vi "Quiz Alt.vi"() -> ()   [LabVIEW 2012]
uses:
  Controls/Quiz Solution.ctl
  Controls/Quiz Question.ctl
  Controls/Problem Type enum.ctl
  Controls/Solution Type enum.ctl
  Controls/Quiz Set Up.ctl
panel:
  in  "Question Array Out":T1[](array[typedef])=[{"Text"="\"Enter \"\"AAA\"\"\"", "Problem Type"=enum."Text", "Solution Type"=enum."Text", "Picture"=bytes[0], "MultiText"=[], "Solution"={"Answer State"=enum."Unanswered", "TF Answer"=enum."No Selection", "Text Answer"="AAA", "Multi Answer"=[], "ExactMatch"=TRUE, "Numeric Answer"={"NumAnswer"=0.0, "Num Sol MAX"=0.0, "Num Sol MIN"=0.0, "SigFig?"=FALSE, "Num Sig Figs"=0}, "T/F_Solution"=FALSE}}, {"Text"="Which one is conductive", "Problem Type"=enum."Text&Image", "Solution Type"=enum."SelectOne", "Picture"=bytes[117294], "MultiText"=["AA", "BB", "CC"], "Solution"={"Answer State"=enum."Unanswered", "TF Answer"=enum."No Selection", "Text Answer"="", "Multi Answer"=[FALSE, TRUE, FALSE], "ExactMatch"=FALSE, "Numeric Answer"={"NumAnswer"=0.0, "Num Sol MAX"=0.0, "Num Sol MIN"=0.0, "SigFig?"=FALSE, "Num Sig Figs"=0}, "T/F_Solution"=FALSE}}, {"Text"="Select the Vowels", "Problem Type"=enum."Text", "Solution Type"=enum."SelectMultiple", "Picture"=bytes[0], "MultiText"=["A'", "B'", "E'", "D'", "U'"], "Solution"={"Answer State"=enum."Unanswered", "TF Answer"=enum."No Selection", "Text Answer"="", "Multi Answer"=[TRUE, FALSE, TRUE, FALSE, TRUE], "ExactMatch"=FALSE, "Numeric Answer"={"NumAnswer"=0.0, "Num Sol MAX"=0.0, "Num Sol MIN"=0.0, "SigFig?"=FALSE, "Num Sig Figs"=0}, "T/F_Solution"=FALSE}}, {"Text"="Select True", "Problem Type"=enum."Text", "Solution Type"=enum."True/False", "Picture"=bytes[0], "MultiText"=[], "Solution"={"Answer State"=enum."Unanswered", "TF Answer"=enum."No Selection", "Text Answer"="", "Multi Answer"=[], "ExactMatch"=FALSE, "Numeric Answer"={"NumAnswer"=0.0, "Num Sol MAX"=0.0, "Num Sol MIN"=0.0, "SigFig?"=FALSE, "Num Sig Figs"=0}, "T/F_Solution"=TRUE}}, {"Text"="8<x<10 (3 sig figs)", "Problem Type"=enum."Text&Image", "Solution Type"=enum."Numeric", "Picture"=bytes[107210], "MultiText"=[], "Solution"={"Answer State"=enum."Unanswered", "TF Answer"=enum."No Selection", "Text Answer"="", "Multi Answer"=[], "ExactMatch"=FALSE, "Numeric Answer"={"NumAnswer"=0.0, "Num Sol MAX"=0.0, "Num Sol MIN"=8.0, "SigFig?"=TRUE, "Num Sig Figs"=3}, "T/F_Solution"=FALSE}}]
  in  "Problem2":T4={"ProblemNum"=0, "Problem Type"={"Text"="", "Image"=bytes[0], "Text&Image"={"Text (&Image)"="", "Image (&text)"=bytes[0]}}, "Solution Type"={"Numeric"=0.0, "String"="", "Multi"={"A"=FALSE, "B"=FALSE, "C"=FALSE, "D"=FALSE, "E"=TRUE}, "Radio"=enum."E", "True/False"=enum."True", "Short Answer"=""}, "Answer Color"=0, "Submit"=FALSE}
  in  "Problem1":T4={"ProblemNum"=0, "Problem Type"={"Text"="", "Image"=bytes[0], "Text&Image"={"Text (&Image)"="", "Image (&text)"=bytes[0]}}, "Solution Type"={"Numeric"=0.0, "String"="", "Multi"={"A"=FALSE, "B"=FALSE, "C"=FALSE, "D"=FALSE, "E"=TRUE}, "Radio"=enum."E", "True/False"=enum."True", "Short Answer"=""}, "Answer Color"=0, "Submit"=FALSE}
  in  "Problem0":T4={"ProblemNum"=0, "Problem Type"={"Text"="", "Image"=bytes[0], "Text&Image"={"Text (&Image)"="", "Image (&text)"=bytes[0]}}, "Solution Type"={"Numeric"=0.0, "String"="", "Multi"={"A"=FALSE, "B"=FALSE, "C"=FALSE, "D"=FALSE, "E"=TRUE}, "Radio"=enum."E", "True/False"=enum."True", "Short Answer"=""}, "Answer Color"=0, "Submit"=FALSE}
  in  "Problem Offset (0)":i32
  in  "? Ref Array":refnum<vi>[](array[refnum])
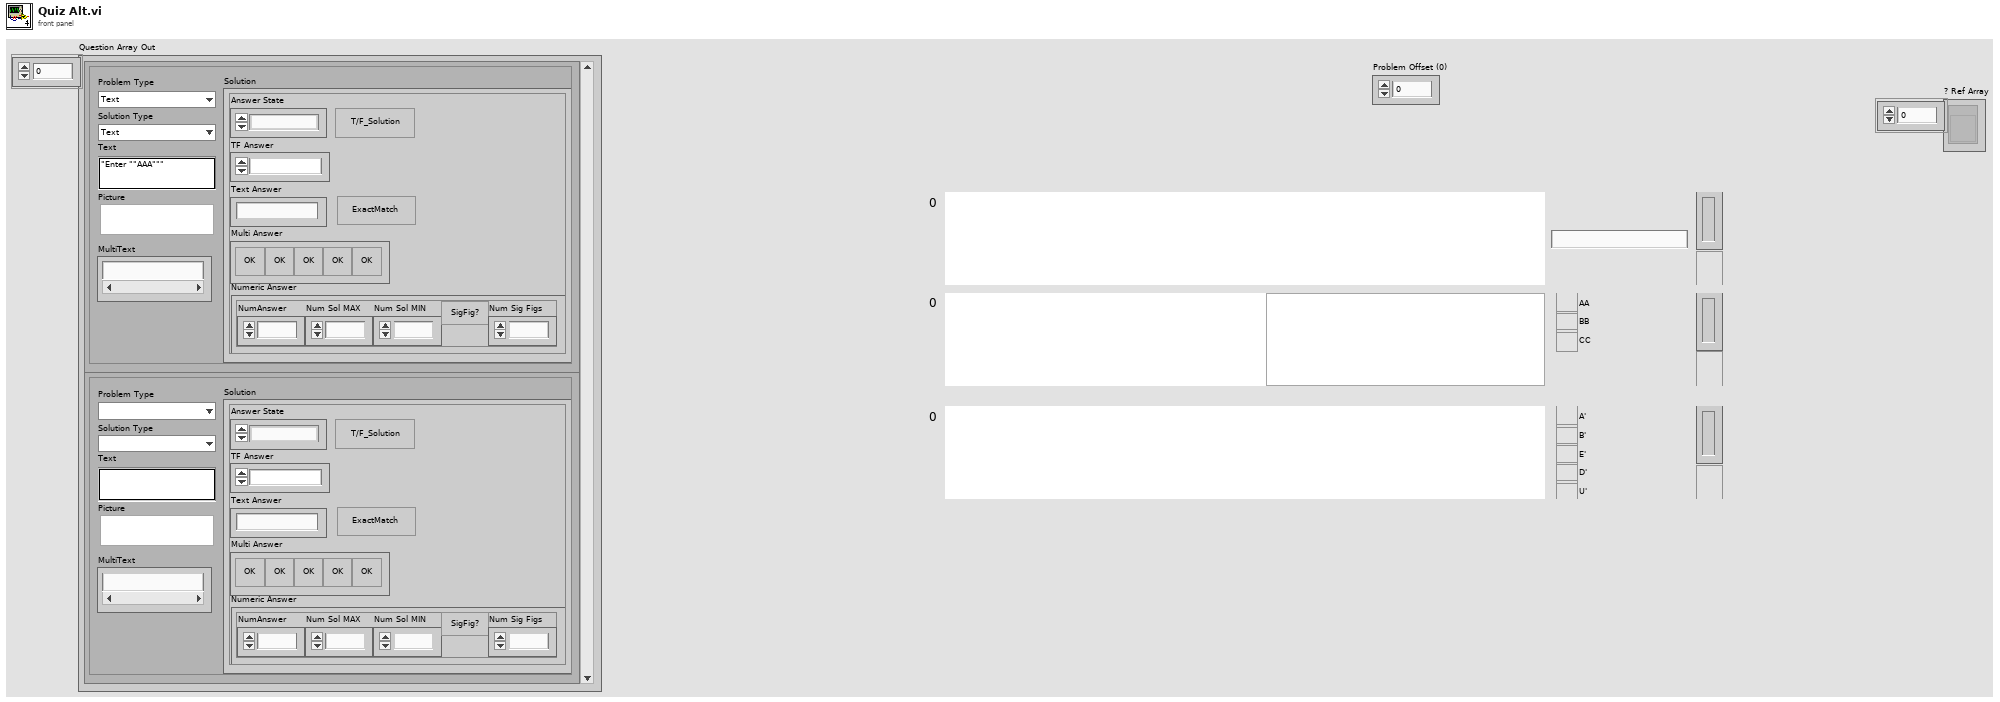
[diagram p1: front panel]
types:
  T1 = typedef "Quiz Set Up.ctl" = cluster{"Text":string, "Problem Type":T2, "Solution Type":T3, "Picture":picture, "MultiText":string[], "Solution":cluster{"Answer State":enum16{"Unanswered", "Correct", "Incorrect"}, "TF Answer":enum32{"No Selection", "True", "False"}, "Text Answer":string, "Multi Answer":bool[], "ExactMatch":bool, "Numeric Answer":cluster{"NumAnswer":dbl, "Num Sol MAX":dbl, "Num Sol MIN":dbl, "SigFig?":bool, "Num Sig Figs":i32}, "T/F_Solution":bool}}
  T2 = typedef "Problem Type enum.ctl" = enum16{"Text", "Image", "Text&Image"}
  T3 = typedef "Solution Type enum.ctl" = enum16{"Numeric", "Text", "SelectMultiple", "SelectOne", "True/False", "ShortAnswer"}
  T4 = typedef "Quiz Question.ctl" = cluster{"ProblemNum":i32, "Problem Type":cluster{"Text":string, "Image":picture, "Text&Image":cluster{"Text (&Image)":string, "Image (&text)":picture}}, "Solution Type":cluster{"Numeric":dbl, "String":string, "Multi":cluster{"A":bool, "B":bool, "C":bool, "D":bool, "E":bool}, "Radio":enum32{"No Selection", "A", "B", "C", "D", "E"}, "True/False":enum32{"No Selection", "True", "False"}, "Short Answer":string}, "Answer Color":u32, "Submit":bool}
  T5 = typedef "Quiz Solution.ctl" = cluster{"Answer State":enum16{"Unanswered", "Correct", "Incorrect"}, "TF Answer":enum32{"No Selection", "True", "False"}, "Text Answer":string, "Multi Answer":bool[], "NumAnswer":dbl}
  T6 = enum8{"Enabled", "Disabled", "Disabled and Grayed Out"}
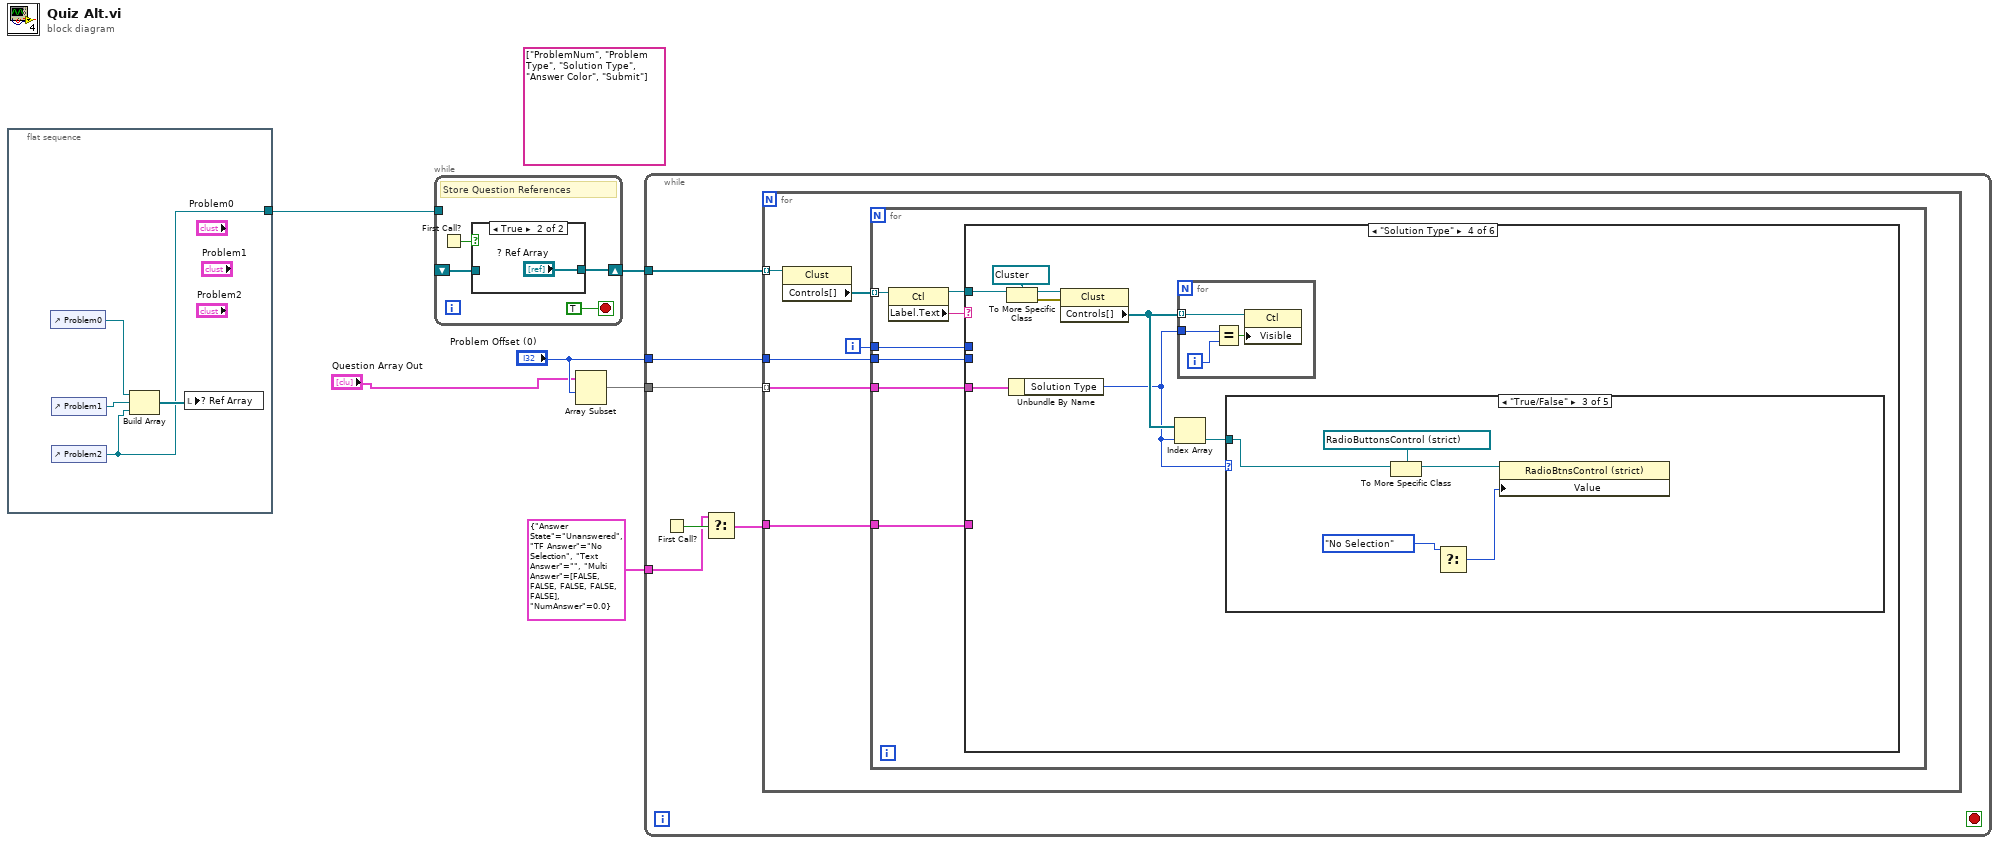
[diagram p0: block diagram]
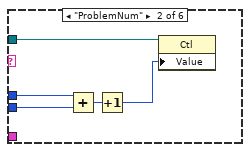
[diagram p3: hidden frame]
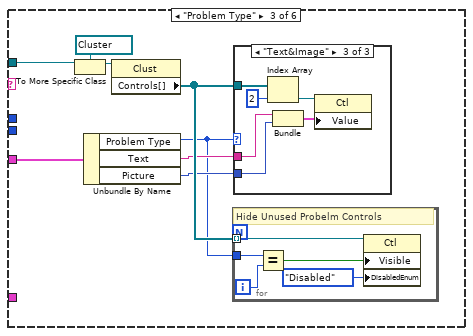
[diagram p4: hidden frame]
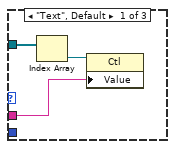
[diagram p5: hidden frame]
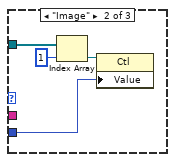
[diagram p6: hidden frame]
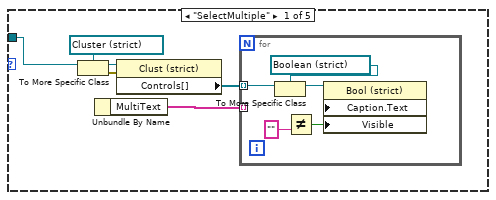
[diagram p7: hidden frame]
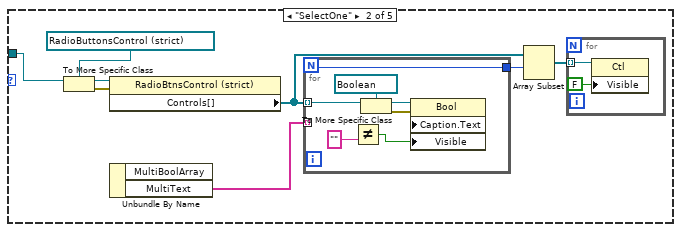
[diagram p8: hidden frame]
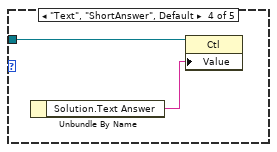
[diagram p9: hidden frame]
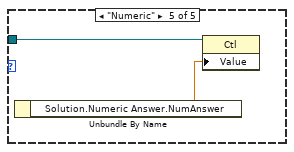
[diagram p10: hidden frame]
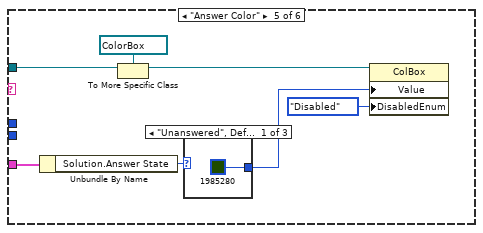
[diagram p11: hidden frame]
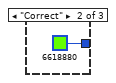
[diagram p12: hidden frame]
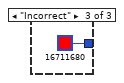
[diagram p13: hidden frame]
diagram:
  (unwired) string[] ["ProblemNum", "Problem Type", "Solution Type", "Answer Color", "Submit"] ("Array")
  n1 = flat-sequence {
    tunnel: [w7] -> w4
    frame #0 {
      n2 = control-ref of="Problem0"() -> (w9:refnum<vi>)
      n3 = control-ref of="Problem1"() -> (w8:refnum<vi>)
      n4 = control-ref of="Problem2"() -> (w7:refnum<vi>)
      n5 = Build Array(w9, w8, w7) -> (w10:refnum<vi>[])
      n6 = local write "? Ref Array"(w10) -> ()
    }
  }
  n7 = while {
    shift-right: [w14] -> w6
    shift-left: _ -> [w13]
    tunnel: w4 -> [_]
    stop <- TRUE stop-if-true
    # "Store Question References"
    n8 = First Call?() -> (First Call?: T/F=w11:bool)
    n9 = case shown="True" w11 {
      tunnel: [w15 "? Ref Array"] -> w14
      tunnel: w13 -> [w15 _]
      frame False {
      }
      frame True {
      }
    }
  }
  n10 = Array Subset(array="Question Array Out", index="Problem Offset (0)") -> (w5:T1[])  [unwired: 1 in]
  n11 = while {
    tunnel: w6 -> [w22]
    tunnel: w5 -> [w21]
    tunnel: "Problem Offset (0)" -> [w20]
    tunnel: T5 {"Answer State"=enum."Unanswered", "TF Answer"=enum."No Selection", "Text Answer"="", "Multi Answer"=[FALSE, FALSE, FALSE, FALSE, FALSE], "NumAnswer"=0.0} ("Solution") -> [w18]
    stop <- _ stop-if-true
    n12 = First Call?() -> (First Call?: T/F=w19:bool)
    n13 = Select(t=w18, s=w19) -> (s? t:f=w17:T5)  [unwired: 1 in]
    n14 = for {
      tunnel: w22 -> [w28] mode=indexing
      tunnel: w21 -> [w24] mode=indexing
      tunnel: w20 -> [w26]
      tunnel: w17 -> [w23]
      i -> [w25]
      n15 = property class="Clust"(reference=w28) -> ("Controls[]"=w27:refnum<vi>[])  [unwired: 1 in, 2 out]
      n16 = for {
        tunnel: w27 -> [w35] mode=indexing
        tunnel: w26 -> [w32]
        tunnel: w25 -> [w31]
        tunnel: w24 -> [w30]
        tunnel: w23 -> [w29]
        n17 = property class="Ctl"(reference=w35) -> (reference out=w33:refnum<vi>, "Label.Text"=w34:string)  [unwired: 1 in, 1 out]
        n18 = case shown="\"Solution Type\"" w34 {
          tunnel: w33 -> [_ w40 w45 w73 w119 _]
          tunnel: w32 -> [_ w38 _ _ _ _]
          tunnel: w31 -> [_ w37 _ _ _ _]
          tunnel: w30 -> [_ _ w48 w67 w122 _]
          tunnel: w29 -> [_ _ _ _ _ _]
          frame "NULL", Default {
          }
          frame "ProblemNum" {
            n19 = Add(x=w37, y=w38) -> (x+y=w39:i32)
            n20 = Increment(x=w39) -> (x+1=w36:i32)
            n21 = property class="Ctl"(reference=w40, "Value"=w36) -> ()  [unwired: 1 in, 2 out]
          }
          frame "Problem Type" {
            n22 = To More Specific Class(target class=refnum<vi> refnum ("Problem Type"), reference=w45) -> (specific class reference=w46:refnum<vi>)  [unwired: 1 in, 1 out]
            n23 = Unbundle By Name(w48) -> ("Problem Type"=w41:T2, "Text"=w43:string, "Picture"=w42:picture)
            n24 = property on="Property Node" class="Clust"(reference=w46) -> ("Controls[]"=w44:refnum<vi>[])  [unwired: 1 in, 2 out]
            n25 = for "Problem Controls" {
              tunnel: w44 -> [w66] mode=indexing
              tunnel: w41 -> [w64]
              i -> [w63]
              # "Hide Unused Probelm Controls"
              n26 = Equal?(x=w64, y=w63) -> (x = y?=w62:bool)
              n27 = property on="Property Node" class="Ctl"(reference=w66, "Visible"=w62, "DisabledEnum"=T6."Disabled" ("Disabled")) -> ()  [unwired: 1 in, 2 out]
            }
            n28 = case shown="\"Text&Image\"" w41 {
              tunnel: w44 -> [w51 w55 w61]
              tunnel: w43 -> [w49 _ w58]
              tunnel: w42 -> [_ w52 w57]
              frame "Text", Default {
                n29 = Index Array(array=w51) -> (element=w50:refnum<vi>)  [unwired: 1 in]
                n30 = property on="Property Node" class="Ctl"(reference=w50, "Value"=w49) -> ()  [unwired: 1 in, 2 out]
              }
              frame "Image" {
                n31 = Index Array(array=w55, index=1) -> (element=w53:refnum<vi>)
                n32 = property on="Property Node" class="Ctl"(reference=w53, "Value"=w52) -> ()  [unwired: 1 in, 2 out]
              }
              frame "Text&Image" {
                n33 = Index Array(array=w61, index=2) -> (element=w59:refnum<vi>)
                n34 = Bundle("Text"=w58, "Picture"=w57) -> (w56:cluster{"Text":string, "Picture":picture})  [unwired: 1 in]
                n35 = property on="Property Node" class="Ctl"(reference=w59, "Value"=w56) -> ()  [unwired: 1 in, 2 out]
              }
            }
          }
          frame "Solution Type" {
            n36 = To More Specific Class(target class=refnum<vi> refnum ("Problem Type"), reference=w73) -> (specific class reference=w72:refnum<vi>, error out=w71:errorcluster)  [unwired: 1 in]
            n37 = Unbundle By Name(w67) -> ("Solution Type"=w69:T3)
            n38 = property on="Property Node" class="Clust"(reference=w72, error in=w71) -> ("Controls[]"=w70:refnum<vi>[])  [unwired: 2 out]
            n39 = Index Array(array=w70, index=w69) -> (element=w68:refnum<vi>)
            n40 = for {
              tunnel: w70 -> [w115] mode=indexing
              tunnel: w69 -> [w113]
              i -> [w112]
              n41 = Equal?(x=w113, y=w112) -> (x = y?=w114:bool)
              n42 = property on="Property Node" class="Ctl"(reference=w115, "Visible"=w114) -> ()  [unwired: 1 in, 2 out]
            }
            n43 = case "Populate Solution Controls" shown="\"True/False\"" w69 {
              tunnel: w68 -> [w75 w86 w105 w109 w110]
              frame "SelectMultiple" {
                n44 = To More Specific Class(target class=refnum<vi> refnum ("Multi"), reference=w75) -> (specific class reference=w80:refnum<vi>, error out=w79:errorcluster)  [unwired: 1 in]
                n45 = Unbundle By Name() -> ("MultiText"=w76:string[])  [unwired: 1 in]
                n46 = property on="Property Node" class="Clust (strict)"(reference=w80, error in=w79) -> ("Controls[]"=w78:refnum<vi>[])  [unwired: 2 out]
                n47 = for {
                  tunnel: w78 -> [w85] mode=indexing
                  tunnel: w76 -> [_] mode=indexing
                  n48 = To More Specific Class(target class=refnum<vi> refnum ("A"), reference=w85) -> (specific class reference=w84:refnum<vi>)  [unwired: 1 in, 1 out]
                  n49 = Not Equal?(y="") -> (x != y?=w82:bool)  [unwired: 1 in]
                  n50 = property on="Property Node" class="Bool (strict)" props=["Caption", "Text", "Visible"](reference=w84, "Visible"=w82) -> ()  [unwired: 2 in, 2 out]
                }
              }
              frame "SelectOne" {
                n51 = To More Specific Class(target class=refnum<vi> refnum ("Radio"), reference=w86) -> (specific class reference=w89:refnum<vi>, error out=w91:errorcluster)  [unwired: 1 in]
                n52 = property on="Property Node" class="RadioBtnsControl (strict)"(reference=w89, error in=w91) -> ("Controls[]"=w92:refnum<vi>[])  [unwired: 2 out]
                n53 = Unbundle By Name() -> ("MultiText"=w87:string[])  [unwired: 1 in, 1 out]
                n54 = for {
                  N -> [w98]
                  tunnel: w87 -> [_] mode=indexing
                  tunnel: w92 -> [w102] mode=indexing
                  tunnel: [w98] -> w93
                  n55 = Not Equal?(y="") -> (x != y?=w96:bool)  [unwired: 1 in]
                  n56 = To More Specific Class(target class=refnum<vi> refnum ("Problem Type"), reference=w102) -> (specific class reference=w101:refnum<vi>, error out=w99:errorcluster)  [unwired: 1 in]
                  n57 = property on="Property Node" class="Bool" props=["Caption", "Text", "Visible"](reference=w101, error in=w99, "Visible"=w96) -> ()  [unwired: 1 in, 2 out]
                }
                n58 = Array Subset(array=w92, index=w93) -> (w90:refnum<vi>[])  [unwired: 1 in]
                n59 = for {
                  tunnel: w90 -> [w94] mode=indexing
                  n60 = property on="Property Node" class="Ctl"(reference=w94, "Visible"=FALSE) -> ()  [unwired: 1 in, 2 out]
                }
              }
              frame "True/False" {
                n61 = To More Specific Class(target class=refnum<vi> refnum ("True/False"), reference=w105) -> (specific class reference=w107:refnum<vi>)  [unwired: 1 in, 1 out]
                n62 = Select(t=enum32{"No Selection", "True", "False"}."No Selection" ("Value")) -> (s? t:f=w103:enum32{"No Selection", "True", "False"})  [unwired: 2 in]
                n63 = property on="Property Node" class="RadioBtnsControl (strict)"(reference=w107, "Value"=w103) -> ()  [unwired: 1 in, 2 out]
              }
              frame "Text", "ShortAnswer", Default {
                n64 = Unbundle By Name() -> ("Solution.Text Answer"=w108:string)  [unwired: 1 in]
                n65 = property on="Property Node" class="Ctl"(reference=w109, "Value"=w108) -> ()  [unwired: 1 in, 2 out]
              }
              frame "Numeric" {
                n66 = Unbundle By Name() -> ("Solution.Numeric Answer.NumAnswer"=w111:dbl)  [unwired: 1 in]
                n67 = property on="Property Node" class="Ctl"(reference=w110, "Value"=w111) -> ()  [unwired: 1 in, 2 out]
              }
            }
          }
          frame "Answer Color" {
            n68 = Unbundle By Name(w122) -> ("Solution.Answer State"=w120:enum16{"Unanswered", "Correct", "Incorrect"})
            n69 = To More Specific Class(target class=refnum<vi> refnum ("Problem Type"), reference=w119) -> (specific class reference=w118:refnum<vi>)  [unwired: 1 in, 1 out]
            n70 = case shown="\"Unanswered\", Default" w120 {
              tunnel: [u32 1985280 u32 6618880 u32 16711680] -> w117
              frame "Unanswered", Default {
              }
              frame "Correct" {
              }
              frame "Incorrect" {
              }
            }
            n71 = property class="ColBox"(reference=w118, "Value"=w117, "DisabledEnum"=T6."Disabled" ("Disabled")) -> ()  [unwired: 1 in, 2 out]
          }
          frame "Submit" {
          }
        }
      }
    }
  }
